vi "one_button.vi"() -> ()   [LabVIEW 2015]
uses:
  <vilib>/rvi/Emulation/niFpgaGetClockAttributes.vi
  <vilib>/rvi/Emulation/niFpgaSctlEmulationGetInTimedLoop.vi
  <vilib>/rvi/Emulation/niFpgaEmulationReportErrorSimple.vi
  <vilib>/rvi/eio/common/nirviEmuTemplateMethod_errors.vi
  <vilib>/rvi/Emulation/niFpgaCriticalErrorInLSC.vi
  <vilib>/eio/EIONode/EIONode.xnode
panel:
  out "x-y 3":i16
  out "x-y 2":i16
  out "x-y":i16
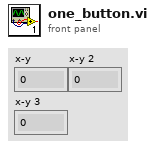
[diagram p1: front panel]
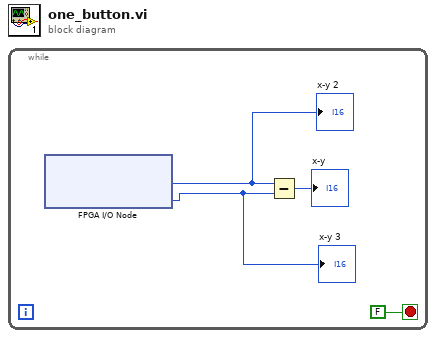
[diagram p0: block diagram]
diagram:
  n1 = while {
    stop <- FALSE stop-if-true
    n2 = xnode "FPGA I/O Node"() -> ("Connector0/AI0"=w3:i16, "Connector0/AI1"=w2:i16)  [unwired: 2 in, 2 out]
    "x-y 2" <- w3
    "x-y 3" <- w2
    n3 = Subtract(x=w3, y=w2) -> (x-y=→"x-y":i16)
  }
